vi "ConvertAllSettings.vi"(3 "data":string="{\"frame_rate\": 199.71975830739089, \"requested_genlock\": 0, \"min_frame_clocks\": 315441, \"is_seq_clk_freq\": 63000000.0, \"pretrigger_frames\": 98, \"edr\": 0, \"duration\": 0.9813751111111112, \"overclock\": 0, \"fpga_temp\": 30, \"requested_horizontal\": 1044, \"frames\": 196, \"requested_multishot_count\": 1, \"requested_pretrigger\": 50, \"requested_edr\": null, \"words_per_frame\": 1848, \"post_trigger_duration\": 0.4906875555555556, \"buffer_end\": 364055, \"dacvrefadc\": 179, \"clocks_per_frame\": 315442, \"requested_duration\": 0.98638199999999998, \"pretrigger\": 50.0, \"multishot_count\": 1, \"posttrigger_frames\": 98, \"vertical\": 672, \"is_temp\": 28, \"requested_vertical\": 676, \"requested_frame_rate\": 199.72, \"requested_force_monochrome\": 0, \"horizontal\": 1040, \"clocks_per_exposure\": 315000, \"digital_gain\": 1.25, \"exposure\": 0.0050000000000000001, \"genlock\": 0, \"pre_trigger_duration\": 0.4906875555555556, \"analog_gain\": 0, \"smart_calibrate\": 0, \"force_monochrome\": 0, \"subsample\": 0, \"requested_exposure\": 0.0050000000000000001, \"iso\": 500, \"requested_iso\": 500, \"requested_overclock\": 0, \"requested_smart_calibrate\": 0, \"requested_subsample\": 0}") -> (1 "Saved Settings:":T1={"Requested Genlock "="0", "Min Frame Clocks "="315441", "Is Seq Clk Freq "="63000000.0", "Pretrigger Frames "="98", "Duration "="0.9813751111111112", "Overclock "="0", "Requested Horizontal "="1044", "Frames "="196", "Requested Pretrigger "="50", "Words per Frame "="1848", "Buffer End "="364055", "Clocks per Frame  "="315442", "Requested Duration "="0.98638199999999998", "Pretrigger "="50.0", "Post-trigger Frames "="98", "Vertical "="672", "Requested Vertical "="676", "Reqested Frame Rate "="199.72", "Frame Rate "="199.71975830739089", "Horizontal "="1040", "Clocks per Exposure "="315000", "Digital Gain "="1.25", "Exposure "="0.0050000000000000001", "Genlock "="0", "Analog Gain "="0", "Subsample "="0", "Requested Exposure "="0.0050000000000000001", "Iso "="500", "Requested Overclock "="0", "Requested Subsample "="0", "Requested Iso"="500", "Multishot"="1", "Requested Multishot"="1", "Monochrome"="0", "Requested mono"="0", "FPGA Temp"="30", "Is Temp"="28", "Posttrigger Duration"="0.4906875555555556", "Pretrigger Duration"="0.4906875555555556", "dacvrefadc"="179"})   [LabVIEW 2015]
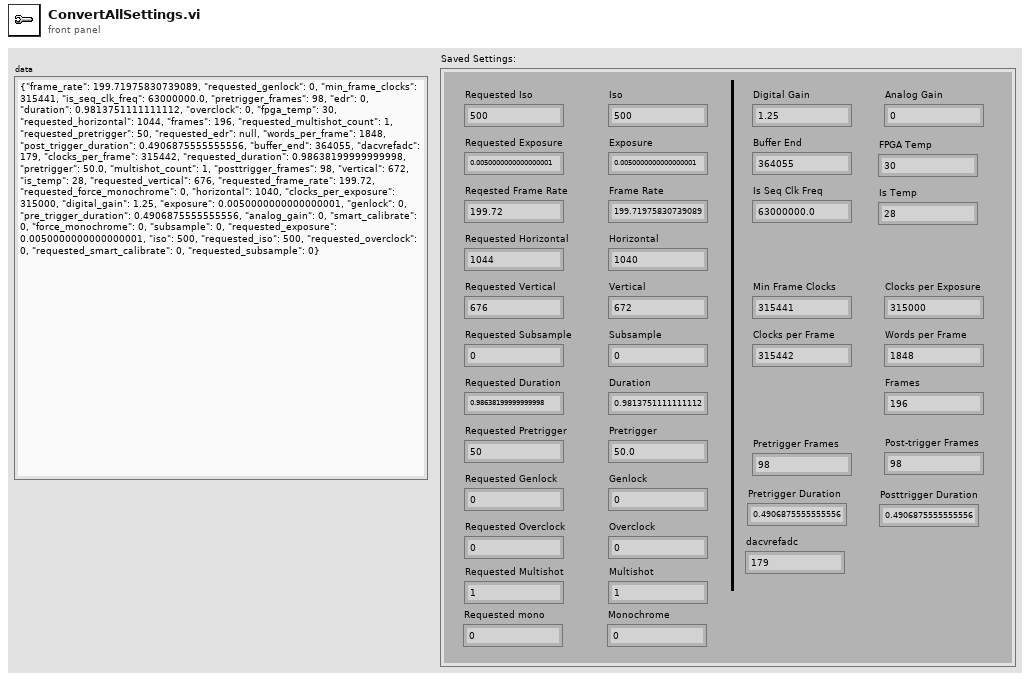
[diagram p1: front panel]
types:
  T1 = cluster{"Requested Genlock ":string, "Min Frame Clocks ":string, "Is Seq Clk Freq ":string, "Pretrigger Frames ":string, "Duration ":string, "Overclock ":string, "Requested Horizontal ":string, "Frames ":string, "Requested Pretrigger ":string, "Words per Frame ":string, "Buffer End ":string, "Clocks per Frame  ":string, "Requested Duration ":string, "Pretrigger ":string, "Post-trigger Frames ":string, "Vertical ":string, "Requested Vertical ":string, "Reqested Frame Rate ":string, "Frame Rate ":string, "Horizontal ":string, "Clocks per Exposure ":string, "Digital Gain ":string, "Exposure ":string, "Genlock ":string, "Analog Gain ":string, "Subsample ":string, "Requested Exposure ":string, "Iso ":string, "Requested Overclock ":string, "Requested Subsample ":string, "Requested Iso":string, "Multishot":string, "Requested Multishot":string, "Monochrome":string, "Requested mono":string, "FPGA Temp":string, "Is Temp":string, "Posttrigger Duration":string, "Pretrigger Duration":string, "dacvrefadc":string}
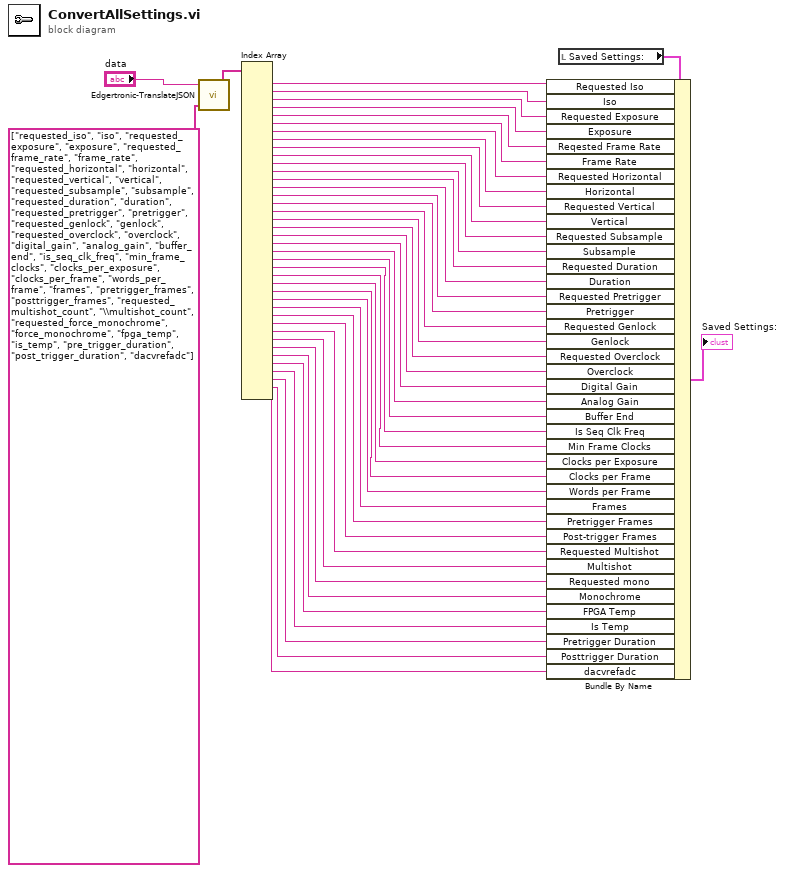
[diagram p0: block diagram]
diagram:
  n1 = call "Edgertronic-TranslateJSON.vi"("Commands"=string[] ["requested_iso", "iso", "requested_exposure", "exposure", "requested_frame_rate", "frame_rate", "requested_horizontal", "horizontal", "requested_vertical", "vertical", "requested_subsample", "subsample", "requested_duration", "duration", "requested_pretrigger", "pretrigger", "requested_genlock", "genlock", "requested_overclock", "overclock", "digital_gain", "analog_gain", "buffer_end", "is_seq_clk_freq", "min_frame_clocks", "clocks_per_exposure", "clocks_per_frame", "words_per_frame", "frames", "pretrigger_frames", "posttrigger_frames", "requested_multishot_count", "\\multishot_count", "requested_force_monochrome", "force_monochrome", "fpga_temp", "is_temp", "pre_trigger_duration", "post_trigger_duration", "dacvrefadc"] ("Array"), "data"="data") -> ("Values"=w8:string[])  [unwired: 3 in]
  n2 = Index Array(array=w8) -> (element #1=w9:string, element #2=w10:string, element #3=w11:string, element #4=w12:string, element #5=w13:string, element #6=w14:string, element #7=w15:string, element #8=w16:string, element #9=w17:string, element #10=w18:string, element #11=w19:string, element #12=w20:string, element #13=w21:string, element #14=w22:string, element #15=w23:string, element #16=w24:string, element #17=w25:string, element #18=w26:string, element #19=w27:string, element #20=w28:string, element #21=w29:string, element #22=w30:string, element #23=w31:string, element #24=w32:string, element #25=w33:string, element #26=w34:string, element #27=w35:string, element #28=w36:string, element #29=w37:string, element #30=w38:string, element #31=w39:string, element #32=w41:string, element #33=w42:string, element #34=w43:string, element #35=w44:string, element #36=w5:string, element #37=w4:string, element #38=w3:string, element #39=w2:string, element #40=w1:string)  [unwired: 40 in]
  n3 = local read "Saved Settings:"() -> (w6:T1)
  n4 = Bundle By Name(cluster=w6, "Requested Iso"=w9, "Iso"=w10, "Requested Exposure"=w11, "Exposure"=w12, "Reqested Frame Rate"=w13, "Frame Rate"=w14, "Requested Horizontal"=w15, "Horizontal"=w16, "Requested Vertical"=w17, "Vertical"=w18, "Requested Subsample"=w19, "Subsample"=w20, "Requested Duration"=w21, "Duration"=w22, "Requested Pretrigger"=w23, "Pretrigger"=w24, "Requested Genlock"=w25, "Genlock"=w26, "Requested Overclock"=w27, "Overclock"=w28, "Digital Gain"=w29, "Analog Gain"=w30, "Buffer End"=w31, "Is Seq Clk Freq"=w32, "Min Frame Clocks"=w33, "Clocks per Exposure"=w34, "Clocks per Frame"=w35, "Words per Frame"=w36, "Frames"=w37, "Pretrigger Frames"=w38, "Post-trigger Frames"=w39, "Requested Multishot"=w41, "Multishot"=w42, "Requested mono"=w43, "Monochrome"=w44, "FPGA Temp"=w5, "Is Temp"=w4, "Pretrigger Duration"=w3, "Posttrigger Duration"=w2, "dacvrefadc"=w1) -> (→"Saved Settings:":T1)
